vi "Log Channels to TDMS.vi"(5 "group name in (Group)":string="Group", 6 "Limit(-1)":i32=-1, 7 "NameRule":T2={"FileNameRule"={"Rule"=enum."Fixed File Name", "Path"=path "", "filename"="data.tdms"}, "FileOperation"=enum."create or replace", "byte order (2:little-endian)"=enum."little-endian", "disable buffering? (T)"=TRUE}, 8 "error in (no error)":errorcluster, 9 "TimeChannel(\"\" Empty to Skip)":string="Time", 10 "Array":variant[](array[variant]), 11 "channel names":string[](array[string])) -> (0 "error out":errorcluster, 1 "DataCount":i32, 2 "File":path)   [LabVIEW 2017]
doc: "Opens a TDMS file and writes the name and type information of every channel in channel names together with the matching values from Array, then closes the file. Limit caps the number of samples per channel, and TimeChannel names the channel used for the time axis (empty to skip it)."
uses:
  _FileName Rule.ctl
  Time/Use Current Time If Input is Empty.vi
  Build FilePath By Rule.vi/7279ca2d-29ef-4966-b9af-d663423eebb9.vi
  Path Type -- Enum.vi
  Make String Safe in Path.vi
  Create Directory if Non-Existant.vi
  <vilib>/Utility/file.llb/Application Directory.vi
  <vilib>/Utility/Data Type/NI_Data Type.lvlib
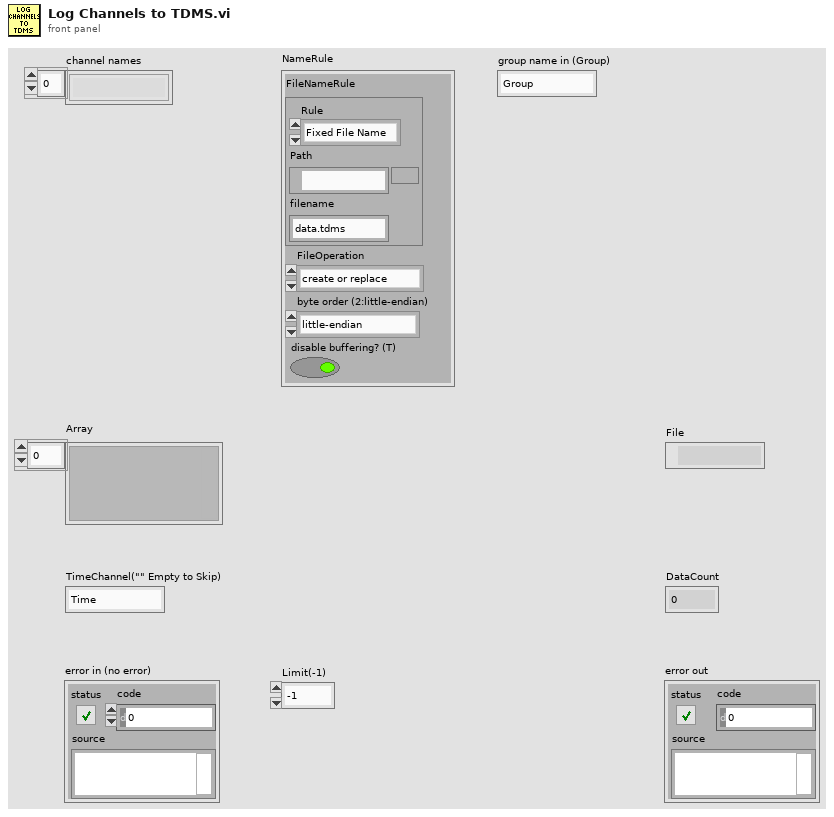
[diagram p1: front panel]
types:
  T1 = typedef "_FileName Rule.ctl" = cluster{"Rule":enum16{"Fixed File Name", "Indexed File Name", "TimeBased File Name"}, "Path":path, "filename":string}
  T2 = cluster{"FileNameRule":T1, "FileOperation":enum16{"open", "open or create", "create or replace", "create", "open (read-only)"}, "byte order (2:little-endian)":enum16{"big-endian, network order", "native, host order", "little-endian"}, "disable buffering? (T)":bool}
  T3 = enum16{"open", "open or create", "create or replace", "create", "open (read-only)"}
  T4 = enum16{"big-endian, network order", "native, host order", "little-endian"}
  T5 = typedef "NI_Data Type.lvlib/Data Type.ctl" = enum8{"Invalid Type", "Void", "I8", "I16", "I32", "I64", "U8", "U16", "U32", "U64", "Single Float", "Double Float", "Extended Float", "Single Complex", "Double Complex", "Extended Complex", "Enum U8", "Enum U16", "Enum U32", "Enum U64", "Single Float With Unit", "Double Float With Unit", "Extended Float With Unit", "Single Complex with Unit", "Double Complex with Unit", "Extended Complex with Unit", "Boolean", "String", "Path", "Picture", "Tag", "Array", "Cluster", "Variant", "LV Variant", "Waveform", "Timestamp", "Digital Waveform", "Digital Data", "ExpressData", "Refnum", "External Data", "VI", "Poly VI", "LabVIEW Class Instance", "Fixed Point"}
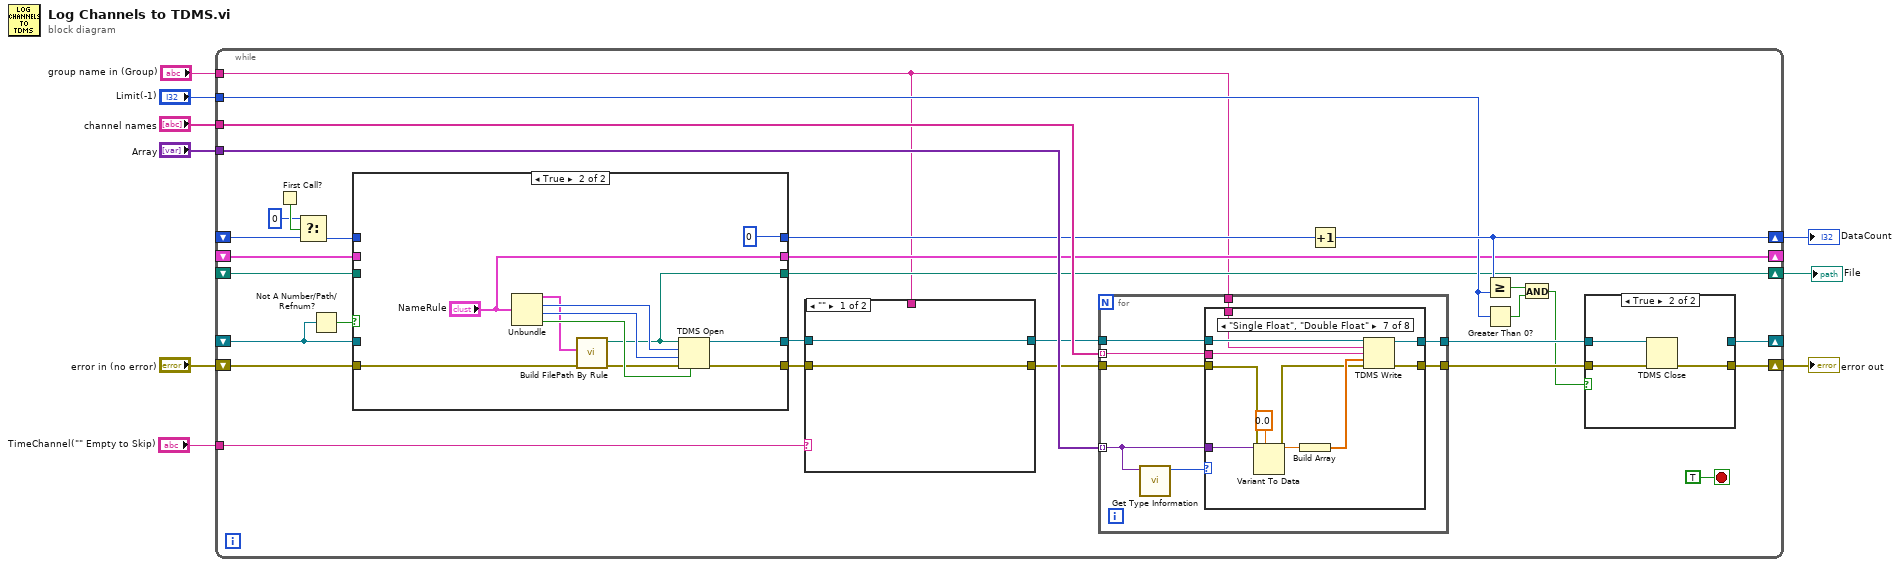
[diagram p0: block diagram]
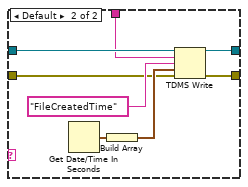
[diagram p2: hidden frame]
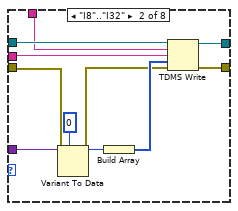
[diagram p4: hidden frame]
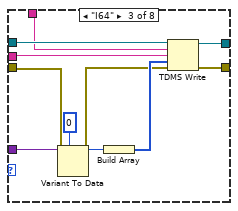
[diagram p5: hidden frame]
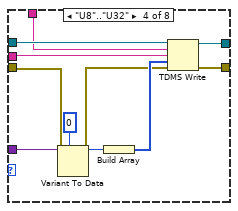
[diagram p6: hidden frame]
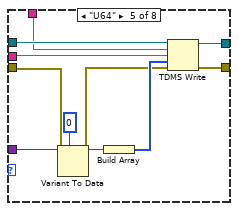
[diagram p7: hidden frame]
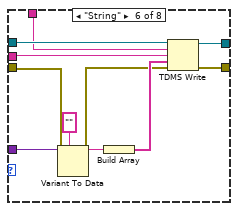
[diagram p8: hidden frame]
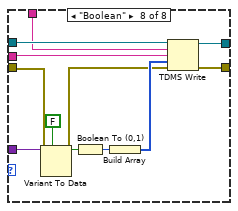
[diagram p9: hidden frame]
diagram:
  n1 = while {
    shift-right: [w39] -> w8
    shift-left: "error in (no error)" -> [w16]
    shift-right: [w38] -> _
    shift-left: _ -> [w36]
    tunnel: "channel names" -> [w34]
    tunnel: "Array" -> [w33]
    shift-right: [w28] -> w4
    shift-left: _ -> [w29]
    tunnel: "Limit(-1)" -> [w26]
    shift-right: [w23] -> w3
    shift-left: _ -> [w22]
    shift-right: [w17] -> _
    shift-left: _ -> [w21]
    tunnel: "TimeChannel(\"\" Empty to Skip)" -> [w11]
    tunnel: "group name in (Group)" -> [w10]
    stop <- TRUE stop-if-true
    n2 = First Call?() -> (First Call?: T/F=w19:bool)
    n3 = Select(t=0, s=w19, f=w29) -> (s? t:f=w20:i32)
    n4 = Not A Number/Path/Refnum?(number/path/refnum=w36) -> (NaN/Path/Refnum?=w37:bool)
    n5 = case shown="True" w37 {
      tunnel: [w147 w150] -> w15
      tunnel: [w146 w149] -> w14
      tunnel: w36 -> [w147 _]
      tunnel: [w145 0] -> w30
      tunnel: w20 -> [w145 _]
      tunnel: [w144 w151] -> w23
      tunnel: w22 -> [w144 _]
      tunnel: w21 -> [w143 _]
      tunnel: [w143 "NameRule"] -> w17
      tunnel: w16 -> [w146 w152]
      frame False {
      }
      frame True {
        n6 = Unbundle("NameRule") -> ("FileNameRule"=w148:T1, "FileOperation"=w154:T3, "byte order (2:little-endian)"=w155:T4, "disable buffering? (T)"=w156:bool)
        n7 = call "Build FilePath By Rule.vi"("error in (no error)"=w152, "FileNameRule"=w148) -> ("error out"=w153:errorcluster, "File"=w151:path)  [unwired: 8 in]
        n8 = TDMS Open(6:w156, 8:w153, 9:w155, 10:w154, 11:w151) -> (0:w149:errorcluster, 3:w150:refnum<k34>)  [unwired: 2 in]
      }
    }
    n9 = case shown="\"\"" w11 {
      tunnel: w15 -> [w41 w46]
      tunnel: w14 -> [w40 w45]
      tunnel: [w41 w44] -> w13
      tunnel: [w40 w43] -> w12
      tunnel: w10 -> [_ w42]
      frame "" {
      }
      frame Default {
        n10 = Get Date/Time In Seconds() -> (seconds since 1Jan1904=w48:timestamp)
        n11 = Build Array(w48) -> (w47:timestamp[])
        n12 = TDMS Write(0:w46, 5:w42, 7:"FileCreatedTime", 9:w47, 11:w45) -> (4:w44:refnum<k34>, 15:w43:errorcluster)  [unwired: 1 in, 2 out]
      }
    }
    n13 = for {
      tunnel: w34 -> [w56] mode=indexing
      tunnel: w33 -> [w51] mode=indexing
      tunnel: w13 -> [w57]
      tunnel: w12 -> [w55]
      tunnel: [w54] -> w32
      tunnel: [w53] -> w31
      tunnel: w10 -> [w52]
      n14 = call <vilib>:"Get Type Information.vi"("Variant"=w51) -> ("Type"=w50:T5)  [unwired: 6 in, 4 out]
      n15 = case shown="\"Single Float\", \"Double Float\"" w50 {
        tunnel: w51 -> [_ w68 w79 w90 w101 w112 w123 w135]
        tunnel: w57 -> [w59 w67 w78 w89 w100 w111 w122 w134]
        tunnel: w56 -> [_ w66 w77 w88 w99 w110 w121 w133]
        tunnel: w55 -> [w58 w62 w73 w84 w95 w106 w117 w129]
        tunnel: [w59 w64 w75 w86 w97 w108 w119 w131] -> w54
        tunnel: [w58 w63 w74 w85 w96 w107 w118 w130] -> w53
        tunnel: w52 -> [_ w60 w71 w82 w93 w104 w115 w126]
        frame Default {
        }
        frame "I8".."I32" {
          n16 = Variant To Data(error in=w62, type=0, Variant=w68) -> (data=w69:i32, error out=w61:errorcluster)
          n17 = Build Array(w69) -> (w65:i32[])
          n18 = TDMS Write(0:w67, 5:w60, 7:w66, 9:w65, 11:w61) -> (4:w64:refnum<k34>, 15:w63:errorcluster)  [unwired: 1 in, 2 out]
        }
        frame "I64" {
          n19 = Variant To Data(error in=w73, type=i64 0, Variant=w79) -> (data=w80:i64, error out=w72:errorcluster)
          n20 = Build Array(w80) -> (w76:i64[])
          n21 = TDMS Write(0:w78, 5:w71, 7:w77, 9:w76, 11:w72) -> (4:w75:refnum<k34>, 15:w74:errorcluster)  [unwired: 1 in, 2 out]
        }
        frame "U8".."U32" {
          n22 = Variant To Data(error in=w84, type=u32 0, Variant=w90) -> (data=w91:u32, error out=w83:errorcluster)
          n23 = Build Array(w91) -> (w87:u32[])
          n24 = TDMS Write(0:w89, 5:w82, 7:w88, 9:w87, 11:w83) -> (4:w86:refnum<k34>, 15:w85:errorcluster)  [unwired: 1 in, 2 out]
        }
        frame "U64" {
          n25 = Variant To Data(error in=w95, type=u64 0, Variant=w101) -> (data=w102:u64, error out=w94:errorcluster)
          n26 = Build Array(w102) -> (w98:u64[])
          n27 = TDMS Write(0:w100, 5:w93, 7:w99, 9:w98, 11:w94) -> (4:w97:refnum<k34>, 15:w96:errorcluster)  [unwired: 1 in, 2 out]
        }
        frame "String" {
          n28 = Variant To Data(error in=w106, type="", Variant=w112) -> (data=w113:string, error out=w105:errorcluster)
          n29 = Build Array(w113) -> (w109:string[])
          n30 = TDMS Write(0:w111, 5:w104, 7:w110, 9:w109, 11:w105) -> (4:w108:refnum<k34>, 15:w107:errorcluster)  [unwired: 1 in, 2 out]
        }
        frame "Single Float", "Double Float" {
          n31 = Variant To Data(error in=w117, type=0.0, Variant=w123) -> (data=w124:dbl, error out=w116:errorcluster)
          n32 = Build Array(w124) -> (w120:dbl[])
          n33 = TDMS Write(0:w122, 5:w115, 7:w121, 9:w120, 11:w116) -> (4:w119:refnum<k34>, 15:w118:errorcluster)  [unwired: 1 in, 2 out]
        }
        frame "Boolean" {
          n34 = Variant To Data(error in=w129, type=FALSE, Variant=w135) -> (data=w136:bool, error out=w128:errorcluster)
          n35 = Boolean To (0,1)(Boolean=w136) -> (0, 1=w127:i16)
          n36 = Build Array(w127) -> (w132:i16[])
          n37 = TDMS Write(0:w134, 5:w126, 7:w133, 9:w132, 11:w128) -> (4:w131:refnum<k34>, 15:w130:errorcluster)  [unwired: 1 in, 2 out]
        }
      }
    }
    n38 = Increment(x=w30) -> (x+1=w28:i32)
    n39 = Greater Or Equal?(x=w28, y=w26) -> (x >= y?=w27:bool)
    n40 = Greater Than 0?(x=w26) -> (x > 0?=w25:bool)
    n41 = And(x=w27, y=w25) -> (x .and. y?=w24:bool)
    n42 = case shown="True" w24 {
      tunnel: w31 -> [w138 w142]
      tunnel: w32 -> [w139 w141]
      tunnel: [w138 w140] -> w39
      tunnel: [w139 _] -> w38
      frame False {
      }
      frame True {
        n43 = TDMS Close(8:w142, 11:w141) -> (0:w140:errorcluster)  [unwired: 1 out]
      }
    }
  }
  "error out" <- w8
  "DataCount" <- w4
  "File" <- w3
